vi "Stop Acquisition.vi"(8 "error in (no error)":errorcluster, 11 "Hardware Configuration In":T1={"Accel-ai0"=FALSE, "Maximum Input"=0.0, "Minimum Input"=0.0, "HW Sample Rate"=0.0, "SW Sample Rate"=0.0, "Number of Samples"=0, "Accel-ai1"=FALSE, "DAQmx Task"="", "Low Pass Filter"={"Upper Cutoff"=350.0, "Lower Cutoff"=350.0, "Order"=350}} {"Low Pass Filter"."Order" min=0 max=10 step=1}) -> (0 "error out":errorcluster)   [LabVIEW 2022 SP3, in "Acquisition.lvlib"]
doc: "Stops the acquisition."
uses:
  Acquisition.lvlib
  AcquisitionFilter.ctl
  FiniteMeasurement-DAQmx/controls/Hardware Configuration.ctl
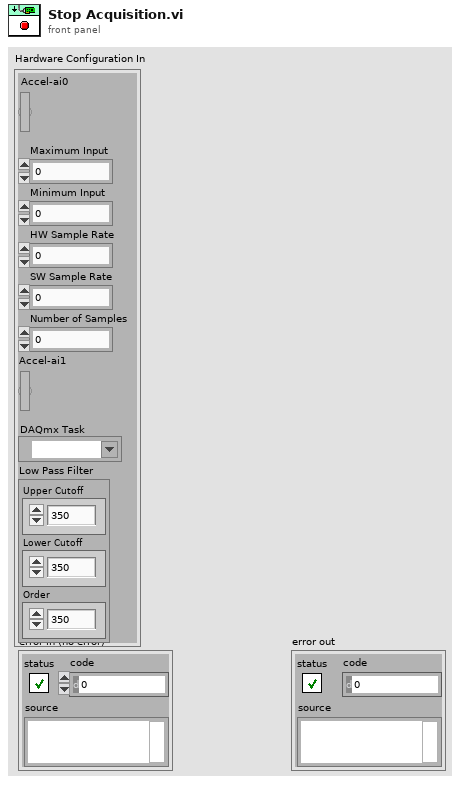
[diagram p1: front panel]
types:
  T1 = typedef "Acquisition.lvlib/Hardware Configuration.ctl" = cluster{"Accel-ai0":bool, "Maximum Input":dbl, "Minimum Input":dbl, "HW Sample Rate":dbl, "SW Sample Rate":dbl, "Number of Samples":i32, "Accel-ai1":bool, "DAQmx Task":refnum<k21>, "Low Pass Filter":T2}
  T2 = typedef "Acquisition.lvlib/AcquisitionFilter.ctl" = cluster{"Upper Cutoff":dbl, "Lower Cutoff":dbl, "Order":i32}
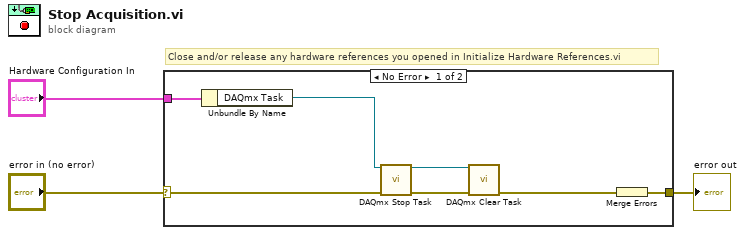
[diagram p0: block diagram]
diagram:
  # "Close and/or release any hardware references you opened in Initialize Hardware References.vi"
  n1 = case shown="No Error" "error in (no error)" {
    selector: "error in (no error)" -> [w8 w11]
    tunnel: [w10 w11] -> w2
    tunnel: "Hardware Configuration In" -> [w9 _]
    frame No Error {
      n2 = Unbundle By Name(w9) -> ("DAQmx Task"=w7:refnum<k21>)
      n3 = call <vilib>:"DAQmx Stop Task.vi"("task/channels in"=w7, "error in"=w8) -> ("task out"=w6:refnum<k21>, "error out"=w5:errorcluster)  [unwired: 12 in]
      n4 = call <vilib>:"DAQmx Clear Task.vi"("task in"=w6, "error in"=w5) -> ("error out"=w4:errorcluster)  [unwired: 13 in]
      n5 = Merge Errors(w4) -> (w10:errorcluster)
    }
    frame Error {
    }
  }
  "error out" <- w2
